vi "Model Initial Values - Add Inports RTM Dependency.vi"(8 "error in (no error)":errorcluster, 9 "Menu hierarchy in":string[](array[string]), 11 "Node Ptr":u64 format="%.0x") -> (0 "error out":errorcluster, 1 "Menu hierarchy out":string[](array[string]), 3 "Action":T1)   [LabVIEW 2011, in "Model Initial Values Custom Device.lvlib"]
uses:
  Model Initial Values Custom Device.lvlib
  <vilib>/NI Veristand/Custom Device API/Custom Device RTM Dependency.ctl
  <vilib>/NI Veristand/Custom Device API/Custom Device API.lvlib
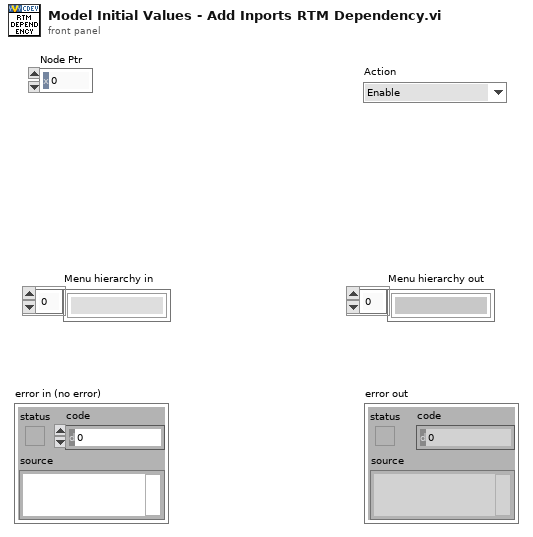
[diagram p1: front panel]
types:
  T1 = typedef "Custom Device API.lvlib/Custom Device RTM Dependency.ctl" = enum16{"Enable", "Disable", "Hide"}
  T2 = typedef "Custom Device API.lvlib/Custom Device Item Ref.ctl" = u64
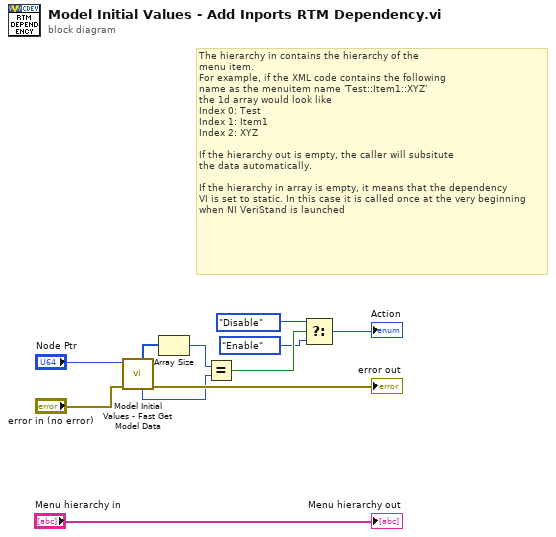
[diagram p0: block diagram]
diagram:
  # "The hierarchy in contains the hierarchy of the\nmenu item.\nFor example, if the XML code contains the following\nname as the menuitem name 'Test::Item1::XYZ'\nthe 1d array would look like\nIndex 0: Test\nIndex 1: Item1\nIndex 2: XYZ\n\nIf the hierarchy out is empty, the caller will subsitute\nthe data automatically.\n\nIf the hierarchy in array is empty, it means that the dependency\nVI is set to static. In this case it is called once at the very beginning\nwhen NI VeriStand is launched"
  n1 = call "Model Initial Values - Fast Get Model Data.vi"("error in (no error)"="error in (no error)", "Local Model Ref in"="Node Ptr") -> ("error out"=→"error out":errorcluster, "Num Inports"=w3:i32, "Inport Refs"=w5:T2[])  [unwired: 4 in, 3 out]
  n2 = Array Size(array=w5) -> (size(s)=w4:i32)
  n3 = Equal?(x=w4, y=w3) -> (x = y?=w8:bool)
  n4 = Select(t=Custom_Device_RTM_Dependency."Disable" ("Action"), s=w8, f=Custom_Device_RTM_Dependency."Enable" ("Action")) -> (s? t:f=→"Action":T1)
  "Menu hierarchy out" <- "Menu hierarchy in"
